vi "Arduino.vi"() -> ()   [LabVIEW 2021]
uses:
  Controls/Arduino-enum.ctl
  <vilib>/MakerHub/LINX/Public/Peripherals/Digital/Digital Read 1 Chan.vi
  <vilib>/MakerHub/LINX/Public/Peripherals/Analog/Analog Read 1 Chan.vi
  <vilib>/MakerHub/LINX/Public/Peripherals/Digital/Digital Write 1 Chan.vi
  <vilib>/MakerHub/LINX/Public/Peripherals/PWM/PWM Set Duty Cycle 1 Chan.vi
  <vilib>/MakerHub/LINX/Public/Peripherals/Digital/Digital Read N Chans.vi
  <vilib>/MakerHub/LINX/Public/Peripherals/Analog/Analog Read N Chans.vi
  <vilib>/MakerHub/LINX/Public/Peripherals/Digital/Digital Write N Chans.vi
  <vilib>/MakerHub/LINX/Private/Local IO/LinxDigitalRead.vi
  <vilib>/MakerHub/LINX/Public/Utilities/Check Channel.vi
  <vilib>/MakerHub/LINX/Private/Local IO/LinxAnalogRead.vi
  <vilib>/MakerHub/LINX/Private/Local IO/LinxDigitalWrite.vi
  <vilib>/MakerHub/LINX/Public/Utilities/Open Serial.vi
  Globals/Global message.vi
  <vilib>/MakerHub/LINX/Public/Peripherals/PWM/PWM Set Duty Cycle N Chans.vi
  <vilib>/MakerHub/LINX/Private/Utilties/Generate Error.vi
  Globals/CH1.vi
  Globals/CH2.vi
  Globals/CH3.vi
  Globals/CH4.vi
  Globals/CH5.vi
  <vilib>/MakerHub/LINX/LMH-LINX.lvlib
panel:
  out "Input value":bool
  in  "DI Channel":u8=13
  in  "Start acquisition":bool
  in  "Output Value":bool
  in  "DO Channel":u8
  in  "Input channel":T1(ring)
  in  "Duty Cycle (0-1)":dbl(slide) scale=0.0..1.0
  in  "PWM Channel":u8=3
  in  "Analog Channel":u8
  in  "Serial Port":refnum<visa-resource-name>="COM3"
  in  "stop":bool
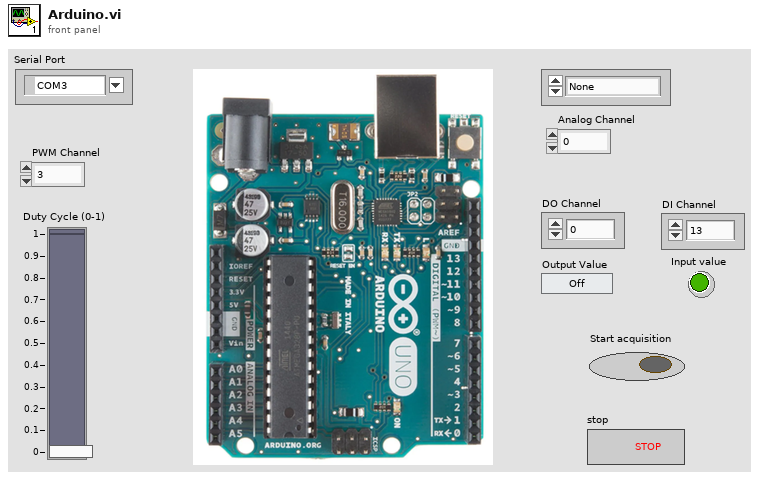
[diagram p1: front panel]
types:
  T1 = enum16{"None", "CH 1", "CH 2", "CH 3", "CH 4", "CH 5"}
  T2 = typedef "Arduino-enum.ctl" = enum16{"Initialize", "Iddle", "Run", "Stop"}
  T3 = typedef "LMH-LINX.lvlib/LINX Ref.ctl" = cluster{"IO":T4, "Interface":T5, "LINX Device Config":T6}
  T4 = typedef "LMH-LINX.lvlib/Platform.ctl" = enum16{"Remote", "Local"}
  T5 = typedef "LMH-LINX.lvlib/Interface.ctl" = enum16{"Serial", "TCP"}
  T6 = typedef "LMH-LINX.lvlib/Device.lvlib/LINX Device Config.ctl" = cluster{"Interface":T5, "COM Port":refnum<visa-resource-name>, "TCP Configuration":T7, "Device Family":u8, "Device ID":u8, "Device Name":string, "TCP Ref":refnum<k5>, "Channels":T8}
  T7 = typedef "LMH-LINX.lvlib/Device.lvlib/TCP Config.ctl" = cluster{"IP Address":string, "Port":u16}
  T8 = typedef "LMH-LINX.lvlib/Channels.ctl" = cluster{"DI":u8[], "DO":u8[], "AI":u8[], "AO":u8[], "PWM":u8[], "QE":u8[], "UART":u8[], "I2C 2":u8[], "SPI":u8[], "CAN":u8[], "Servo":u8[], "AI Ref (V)":dbl, "AI Resolution (Bits)":u8, "AO Ref (V)":dbl, "AO Resolution (Bits)":u8}
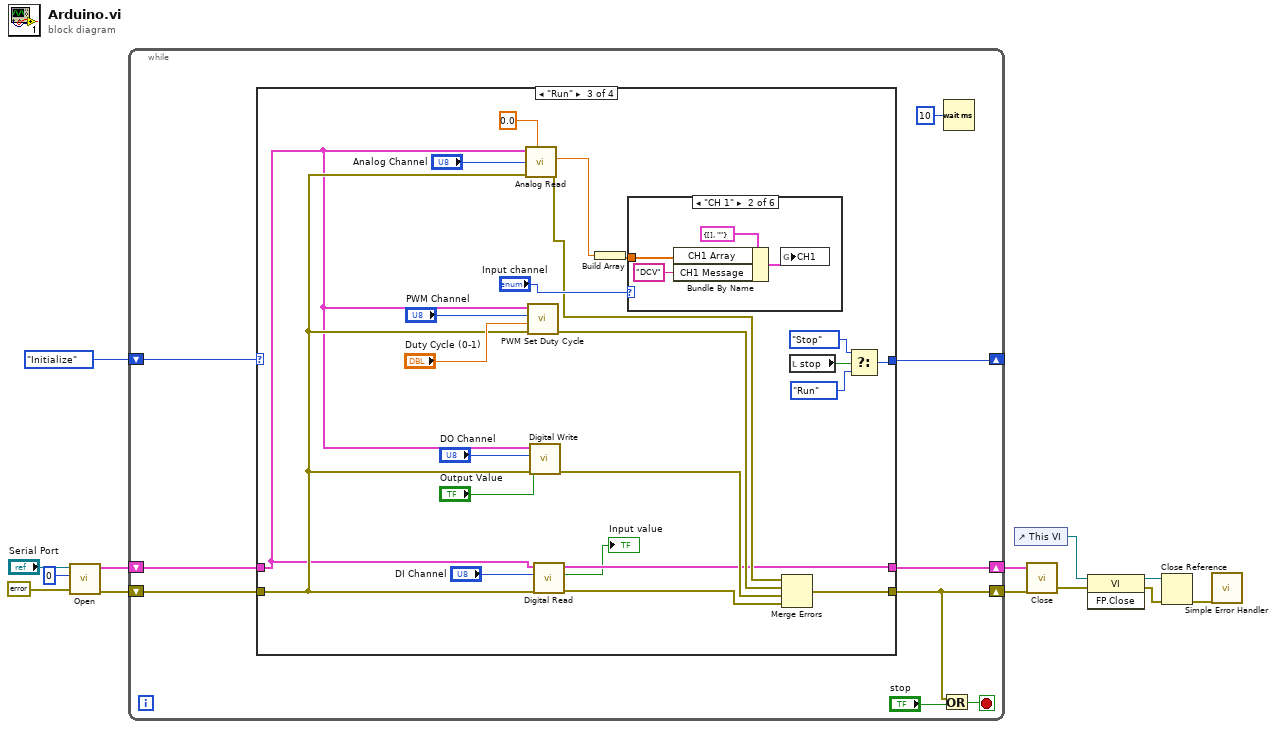
[diagram p0: block diagram]
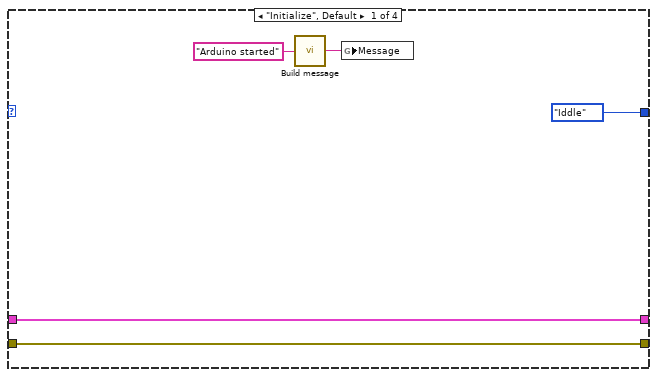
[diagram p2: hidden frame]
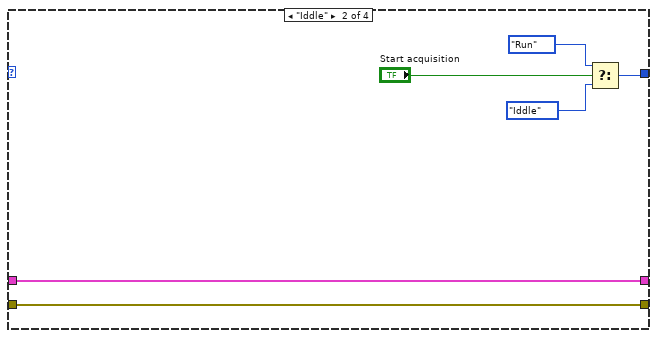
[diagram p3: hidden frame]
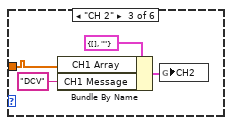
[diagram p5: hidden frame]
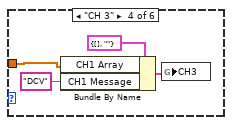
[diagram p6: hidden frame]
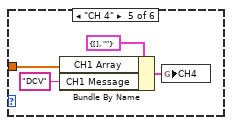
[diagram p7: hidden frame]
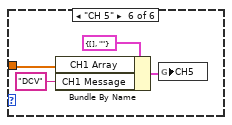
[diagram p8: hidden frame]
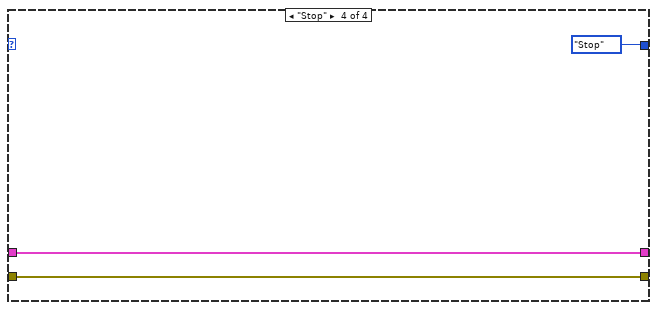
[diagram p9: hidden frame]
diagram:
  n1 = call-poly <vilib>:"Open.vi"("Error In"=errorcluster {"status"=FALSE, "code"=0, "source"=""}, "Baud Rate Override"=u32 0, "Serial Port"="Serial Port") -> ("Error Out"=w8:errorcluster, "LINX Resource"=w9:T3)  [unwired: 6 in, 1 out]
  n2 = while {
    shift-right: [w19] -> _
    shift-left: Arduino-enum."Initialize" ("Enum") -> [w22]
    shift-right: [w15] -> w1
    shift-left: w9 -> [w21]
    shift-right: [w16] -> w2
    shift-left: w8 -> [w20]
    stop <- w18 stop-if-true
    n3 = case shown="\"Run\"" w22 {
      tunnel: w21 -> [w23 w32 w36 w78]
      tunnel: w20 -> [w24 w33 w38 w77]
      tunnel: [Arduino-enum."Iddle" ("Enum") w29 w55 Arduino-enum."Stop" ("Enum")] -> w19
      tunnel: [w24 w33 w40 w77] -> w16
      tunnel: [w23 w32 w35 w78] -> w15
      frame "Initialize", Default {
        n4 = call "Build message.vi"("Input string"="Arduino started") -> ("Output string"=w27:string)
        n5 = global write "Global message.vi" "Message"(w27) -> ()
      }
      frame "Iddle" {
        n6 = Select(t=Arduino-enum."Run" ("Enum"), s="Start acquisition", f=Arduino-enum."Iddle" ("Enum")) -> (s? t:f=w29:T2)
      }
      frame "Run" {
        n7 = call-poly <vilib>:"Analog Read.vi"("Analog Ref Override (V)"=0.0, "Error In"=w38, "Analog Channel"="Analog Channel", "LINX Resource"=w36) -> ("Error Out"=w43:errorcluster, "Voltage"=w49:dbl)  [unwired: 4 in, 2 out]
        n8 = call-poly <vilib>:"PWM Set Duty Cycle.vi"("Error In"=w38, "Duty Cycle (0-1)"="Duty Cycle (0-1)", "PWM Channel"="PWM Channel", "LINX Resource"=w36) -> ("Error Out"=w42:errorcluster)  [unwired: 6 in, 1 out]
        n9 = call-poly <vilib>:"Digital Write.vi"("Error In"=w38, "Output Value"="Output Value", "DO Channel"="DO Channel", "LINX Resource"=w36) -> ("Error Out"=w41:errorcluster)  [unwired: 6 in, 1 out]
        n10 = call-poly <vilib>:"Digital Read.vi"("Error In"=w38, "DI Channel"="DI Channel", "LINX Resource"=w36) -> ("Error Out"=w37:errorcluster, "DI Value"=→"Input value":bool, "LINX Resource"=w35:T3)  [unwired: 6 in]
        n11 = Build Array(w49) -> (w48:dbl[])
        n12 = case shown="\"CH 1\"" "Input channel" {
          tunnel: w48 -> [_ w59 w62 w66 w70 w74]
          frame "None", Default {
          }
          frame "CH 1" {
            n13 = Bundle By Name(cluster=cluster{"CH1 Array":dbl[], "CH1 Message":string} {"CH1 Array"=[], "CH1 Message"=""} ("CH1"), "CH1 Array"=w59, "CH1 Message"="DCV") -> (w58:cluster{"CH1 Array":dbl[], "CH1 Message":string})
            n14 = global write "CH1.vi" "CH1"(w58) -> ()
          }
          frame "CH 2" {
            n15 = Bundle By Name(cluster=cluster{"CH1 Array":dbl[], "CH1 Message":string} {"CH1 Array"=[], "CH1 Message"=""} ("CH1"), "CH1 Array"=w62, "CH1 Message"="DCV") -> (w61:cluster{"CH1 Array":dbl[], "CH1 Message":string})
            n16 = global write "CH2.vi" "CH2"(w61) -> ()
          }
          frame "CH 3" {
            n17 = Bundle By Name(cluster=cluster{"CH1 Array":dbl[], "CH1 Message":string} {"CH1 Array"=[], "CH1 Message"=""} ("CH1"), "CH1 Array"=w66, "CH1 Message"="DCV") -> (w65:cluster{"CH1 Array":dbl[], "CH1 Message":string})
            n18 = global write "CH3.vi" "CH3"(w65) -> ()
          }
          frame "CH 4" {
            n19 = Bundle By Name(cluster=cluster{"CH1 Array":dbl[], "CH1 Message":string} {"CH1 Array"=[], "CH1 Message"=""} ("CH1"), "CH1 Array"=w70, "CH1 Message"="DCV") -> (w69:cluster{"CH1 Array":dbl[], "CH1 Message":string})
            n20 = global write "CH4.vi" "CH4"(w69) -> ()
          }
          frame "CH 5" {
            n21 = Bundle By Name(cluster=cluster{"CH1 Array":dbl[], "CH1 Message":string} {"CH1 Array"=[], "CH1 Message"=""} ("CH1"), "CH1 Array"=w74, "CH1 Message"="DCV") -> (w73:cluster{"CH1 Array":dbl[], "CH1 Message":string})
            n22 = global write "CH5.vi" "CH5"(w73) -> ()
          }
        }
        n23 = Merge Errors(w43, w42, w41, w37) -> (w40:errorcluster)
        n24 = local read "stop"() -> (w53:bool)
        n25 = Select(t=Arduino-enum."Stop" ("Enum"), s=w53, f=Arduino-enum."Run" ("Enum")) -> (s? t:f=w55:T2)
      }
      frame "Stop" {
      }
    }
    n26 = Or(x=w16, y="stop") -> (x .or. y?=w18:bool)
    n27 = Wait (ms)(milliseconds to wait=u32 10) -> ()  [unwired: 1 out]
  }
  n28 = control-ref of="This VI"() -> (w4:refnum<vi>)
  n29 = call <vilib>:"Close.vi"("Error In"=w2, "LINX Resource"=w1) -> ("Error Out"=w7:errorcluster)  [unwired: 9 in]
  n30 = invoke class="VI" method="FP.Close"(reference=w4, error in=w7) -> (reference out=w6:refnum<vi>, error out=w5:errorcluster)  [unwired: 1 in, 1 out]
  n31 = Close Reference(reference=w6, error in (no error)=w5) -> (error out=w3:errorcluster)
  n32 = call <vilib>:"Simple Error Handler.vi"("error in (no error)"=w3) -> ()  [unwired: 4 in, 5 out]
